vi "set_free_amplitude.vi"(8 "error in":errorcluster, 11 "Coarse Approach in":refnum<class "Coarse Approach.lvclass">) -> (0 "error out":errorcluster, 3 "Coarse Approach out":refnum<class "Coarse Approach.lvclass">)   [LabVIEW 2020, in "Coarse Approach.lvclass"]
uses:
  Coarse Approach.lvclass
  Coarse Approach.lvclass/Coarse Approach.ctl
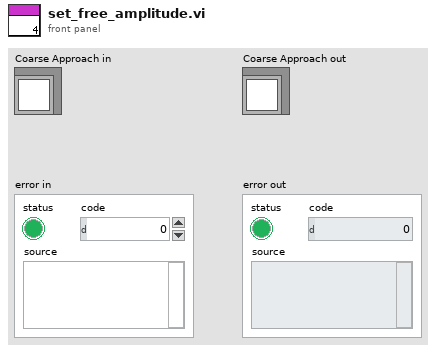
[diagram p1: front panel]
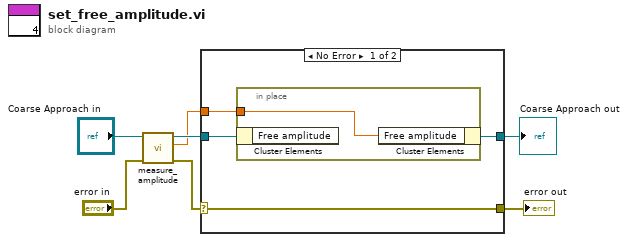
[diagram p0: block diagram]
diagram:
  n1 = call "measure_amplitude.vi"("error in"="error in", "Coarse Approach in"="Coarse Approach in") -> ("error out"=w2:errorcluster, "Amplitude mean"=w4:dbl, "Coarse Approach out"=w5:refnum<class "Coarse Approach.lvclass">)  [unwired: 6 in, 1 out]
  n2 = case shown="No Error" w2 {
    selector: w2 -> [w8 w13]
    tunnel: w5 -> [w11 w14]
    tunnel: w4 -> [w10 _]
    tunnel: [w9 w14] -> w3
    tunnel: [w8 w13] -> w1
    frame No Error {
      n3 = in-place {
        in-place-border: w10 -> [w12]
        n4 = in-place-cluster #1(w11) -> ()  [unwired: 1 out]
        n5 = in-place-cluster #1("Free amplitude"=w12) -> (w9:refnum<class "Coarse Approach.lvclass">)
      }
    }
    frame Error {
    }
  }
  "Coarse Approach out" <- w3
  "error out" <- w1
